vi "Workspace.UI.DisableState.Set.vi"(7 "Enable?":bool=TRUE, 8 "error in (no error)":errorcluster, 11 "State Variables in":T1) -> (0 "error out":errorcluster, 3 "State Variables out":T1)   [LabVIEW 2019, in "Diagnostics Addon Shared.lvlib"]
uses:
  Diagnostics Addon Shared.lvlib
  Types/Workspace.State.ctl
  Types/UI.Refs.ctl
  Types/Command.ctl
  <vilib>/NI VeriStand/Display Template Support/DisplayTemplateSupport.llb/enum_Display Template Handler Minimal To Workspace.ctl
  Types/Workspace.SavedState.ctl
  NationalInstruments.VeriStand.SystemStorage
  <vilib>/NI VeriStand/Execution/Workspace/WorkspaceAPI.ctl
  NationalInstruments.VeriStand.ClientAPI
  <vilib>/NI VeriStand/Display Template Support/DisplayTemplateSupport.llb/enum_Display Template Handler Minimal To Widget Msg.ctl
  <vilib>/NI VeriStand/Execution/Workspace/SystemStateRegEventRef.ctl
  <vilib>/NI VeriStand/Execution/Workspace/Target State Info.ctl
  <vilib>/NI VeriStand/Execution/Workspace/Target State.ctl
  <vilib>/NI VeriStand/Execution/Workspace/SystemStateEventRef.ctl
  Types/Protocol.ctl
  <vilib>/NI VeriStand/Execution/Workspace/NI_VS Workspace ExecutionAPI.lvlib
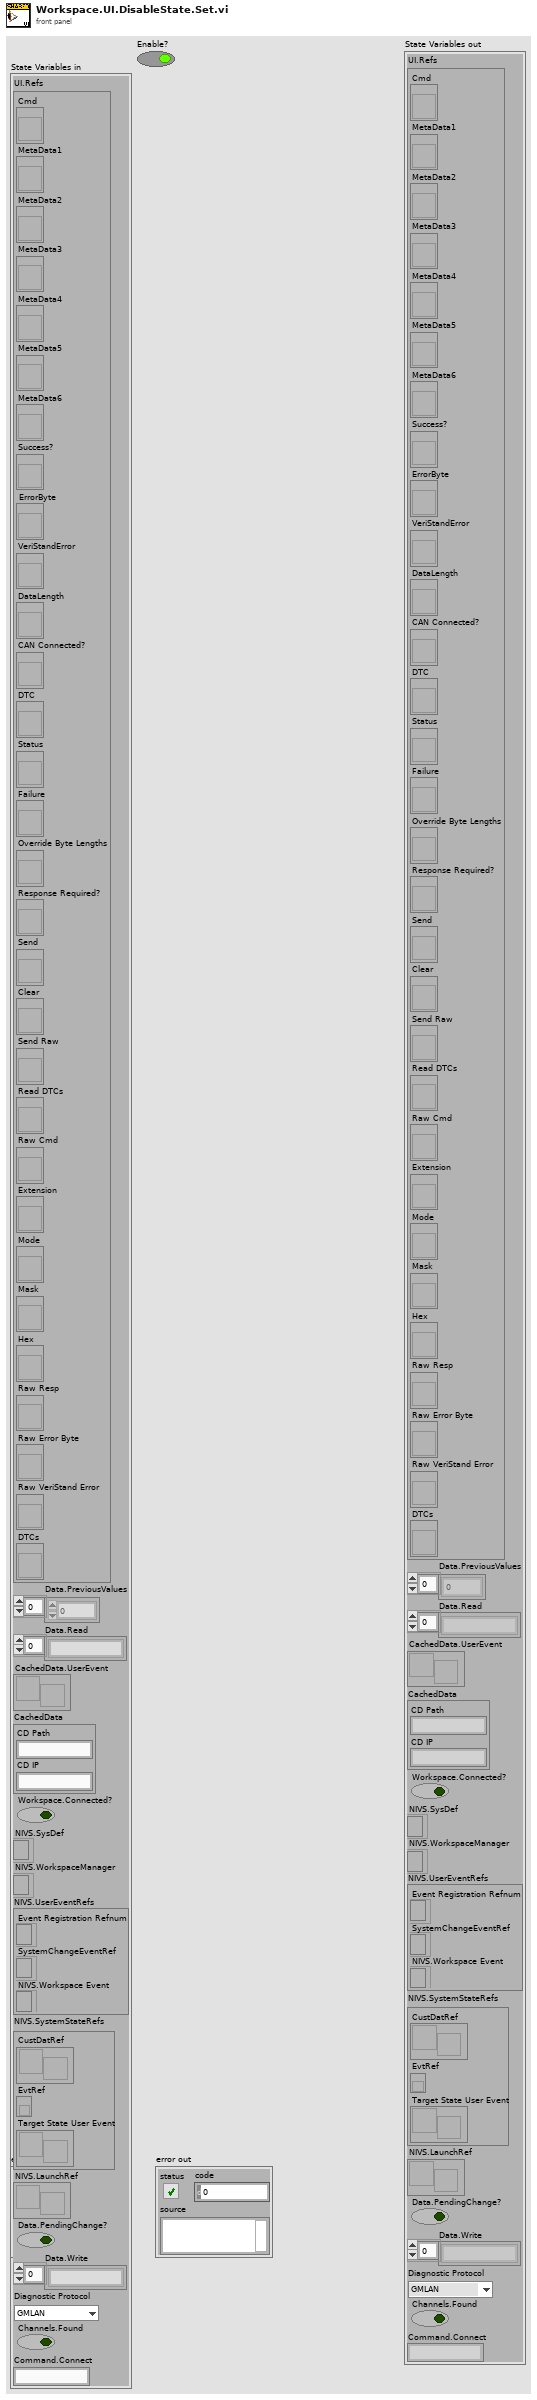
[diagram p1: front panel]
types:
  T1 = typedef "Diagnostics Addon Shared.lvlib/Workspace.State.ctl" = cluster{"UI.Refs":T2, "Data.PreviousValues":dbl[], "Data.Read":string[], "CachedData.UserEvent":refnum<user-event>, "CachedData":T3, "Workspace.Connected?":bool, "NIVS.SysDef":refnum<k24>, "NIVS.WorkspaceManager":T4, "NIVS.UserEventRefs":cluster{"Event Registration Refnum":refnum<event-registration>, "SystemChangeEventRef":T5, "NIVS.Workspace Event":refnum<event-registration>}, "NIVS.SystemStateRefs":T6, "NIVS.LaunchRef":refnum<user-event>, "Data.PendingChange?":bool, "Data.Write":string[], "Diagnostic Protocol":T7, "Channels.Found":bool, "Command.Connect":string}
  T2 = typedef "Diagnostics Addon Shared.lvlib/UI.Refs.ctl" = cluster{"Cmd":refnum<vi>, "MetaData1":refnum<vi>, "MetaData2":refnum<vi>, "MetaData3":refnum<vi>, "MetaData4":refnum<vi>, "MetaData5":refnum<vi>, "MetaData6":refnum<vi>, "Success?":refnum<vi>, "ErrorByte":refnum<vi>, "VeriStandError":refnum<vi>, "DataLength":refnum<vi>, "CAN Connected?":refnum<vi>, "DTC":refnum<vi>, "Status":refnum<vi>, "Failure":refnum<vi>, "Override Byte Lengths":refnum<vi>, "Response Required?":refnum<vi>, "Send":refnum<vi>, "Clear":refnum<vi>, "Send Raw":refnum<vi>, "Read DTCs":refnum<vi>, "Raw Cmd":refnum<vi>, "Extension":refnum<vi>, "Mode":refnum<vi>, "Mask":refnum<vi>, "Hex":refnum<vi>, "Raw Resp":refnum<vi>, "Raw Error Byte":refnum<vi>, "Raw VeriStand Error":refnum<vi>, "DTCs":refnum<vi>}
  T3 = typedef "Diagnostics Addon Shared.lvlib/Workspace.SavedState.ctl" = cluster{"CD Path":string, "CD IP":string}
  T4 = typedef "NI_VS Workspace ExecutionAPI.lvlib/WorkspaceAPI.ctl" = refnum<k24>
  T5 = typedef "NI_VS Workspace ExecutionAPI.lvlib/SystemStateRegEventRef.ctl" = refnum<event-registration>
  T6 = typedef "NI_VS Workspace ExecutionAPI.lvlib/SystemStateEventRef.ctl" = cluster{"CustDatRef":refnum<user-event>, "EvtRef":refnum<k27>, "Target State User Event":refnum<user-event>}
  T7 = typedef "Diagnostics Addon Shared.lvlib/Protocol.ctl" = enum16{"GMLAN", "KWP-2000", "UDS", "User-Defined"}
  T8 = enum8{"Enabled", "Disabled", "Disabled and Grayed Out"}
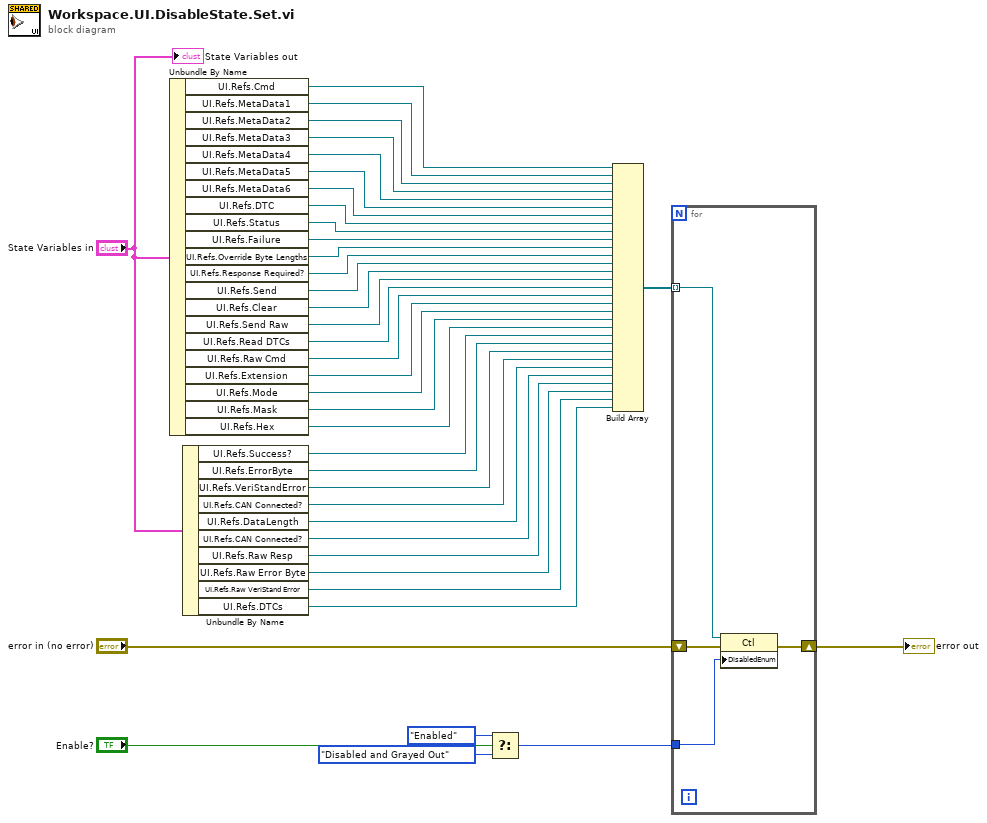
[diagram p0: block diagram]
diagram:
  n1 = Unbundle By Name("State Variables in") -> ("UI.Refs.Cmd"=w17:refnum<vi>, "UI.Refs.MetaData1"=w18:refnum<vi>, "UI.Refs.MetaData2"=w19:refnum<vi>, "UI.Refs.MetaData3"=w20:refnum<vi>, "UI.Refs.MetaData4"=w21:refnum<vi>, "UI.Refs.MetaData5"=w22:refnum<vi>, "UI.Refs.MetaData6"=w23:refnum<vi>, "UI.Refs.DTC"=w24:refnum<vi>, "UI.Refs.Status"=w25:refnum<vi>, "UI.Refs.Failure"=w26:refnum<vi>, "UI.Refs.Override Byte Lengths"=w27:refnum<vi>, "UI.Refs.Response Required?"=w28:refnum<vi>, "UI.Refs.Send"=w29:refnum<vi>, "UI.Refs.Clear"=w30:refnum<vi>, "UI.Refs.Send Raw"=w31:refnum<vi>, "UI.Refs.Read DTCs"=w32:refnum<vi>, "UI.Refs.Raw Cmd"=w33:refnum<vi>, "UI.Refs.Extension"=w34:refnum<vi>, "UI.Refs.Mode"=w35:refnum<vi>, "UI.Refs.Mask"=w36:refnum<vi>, "UI.Refs.Hex"=w12:refnum<vi>)
  n2 = Unbundle By Name("State Variables in") -> ("UI.Refs.Success?"=w10:refnum<vi>, "UI.Refs.ErrorByte"=w9:refnum<vi>, "UI.Refs.VeriStandError"=w8:refnum<vi>, "UI.Refs.CAN Connected?"=w7:refnum<vi>, "UI.Refs.DataLength"=w6:refnum<vi>, "UI.Refs.CAN Connected?"=w5:refnum<vi>, "UI.Refs.Raw Resp"=w4:refnum<vi>, "UI.Refs.Raw Error Byte"=w3:refnum<vi>, "UI.Refs.Raw VeriStand Error"=w2:refnum<vi>, "UI.Refs.DTCs"=w1:refnum<vi>)
  n3 = Select(t=T8."Enabled" ("Disabled"), s="Enable?", f=T8."Disabled and Grayed Out" ("Disabled")) -> (s? t:f=w13:T8)
  n4 = Build Array(w17, w18, w19, w20, w21, w22, w23, w24, w25, w26, w27, w28, w29, w30, w31, w32, w33, w34, w35, w36, w12, w10, w9, w8, w7, w6, w5, w4, w3, w2, w1) -> (w37:refnum<vi>[])
  n5 = for {
    tunnel: w37 -> [w42] mode=indexing
    shift-right: [w41] -> w39
    shift-left: "error in (no error)" -> [w43]
    tunnel: w13 -> [w40]
    n6 = property class="Ctl"(reference=w42, error in=w43, "DisabledEnum"=w40) -> (error out=w41:errorcluster)  [unwired: 1 out]
  }
  "error out" <- w39
  "State Variables out" <- "State Variables in"
